vi "UDT_shutdownTest_UserEventsFGV.vi"() -> (3 "Unit Test Framework Results":T1)   [LabVIEW 2017]
doc: "Use this template to create a user-defined test VI. Define your test requirements and wire the results to the <b>Result (Test)</b> control. Do not modify the <b>Unit Test Framework Results</b> indicator."
uses:
  <vilib>/utf/common/utf_test_result_troll.ctl
  <vilib>/utf/common/utf_test_result.ctl
  <vilib>/utf/common/utf_test_result_failure.ctl
  <vilib>/utf/common/utf_test_comparison_operators.ctl
  <vilib>/utf/common/utf_vi_tag.ctl
  RT/UEFGV/Type Def/UEFGV_States.ctl
  <vilib>/Control Software Solutions Ltd/UTF Helper/SubVIs/UTF Boolean Equals.vi
  <vilib>/Control Software Solutions Ltd/UTF Helper/Unit Test Helper.lvlib
  <vilib>/utf/NI_UnitTestFramework.lvlib
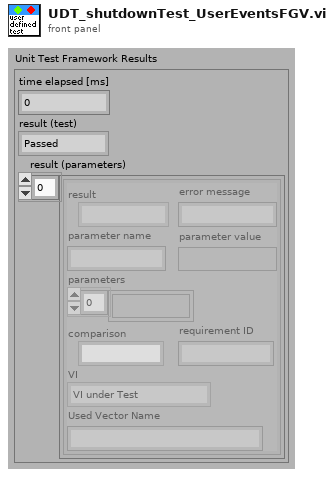
[diagram p1: front panel]
types:
  T1 = typedef "NI_UnitTestFramework.lvlib/utf_test_result_troll.ctl" = cluster{"time elapsed [ms]":u32, "result (test)":T2, "result (parameters)":T3[]}
  T2 = typedef "NI_UnitTestFramework.lvlib/utf_test_result.ctl" = enum16{"Passed", "Failed", "Error", "Skipped", "Not Processed"}
  T3 = typedef "NI_UnitTestFramework.lvlib/utf_test_result_failure.ctl" = cluster{"result":T2, "error message":string, "parameter name":string, "parameter value":variant, "parameters":variant[], "comparison":T4, "requirement ID":string, "VI":T5, "Used Vector Name":string}
  T4 = typedef "NI_UnitTestFramework.lvlib/utf_test_comparison_operators.ctl" = enum16{"=", "!=", ">", ">=", "<", "<=", "range", "symmetric tolerance", "asymmetric tolerance", "string contains", "string not contain", "array size", "string length", "array range", "by element", "array range (limit array)", "user-defined", "array contains", "array not contain", "vector length", "= (elm)", "!= (elm)", "= (case insensitive)", "!= (case insensitive)"}
  T5 = typedef "NI_UnitTestFramework.lvlib/utf_vi_tag.ctl" = enum16{"Setup VI", "VI under Test", "Teardown VI"}
  T6 = typedef "UEFGV_States.ctl" = enum16{"Create", "Get", "Destroy"}
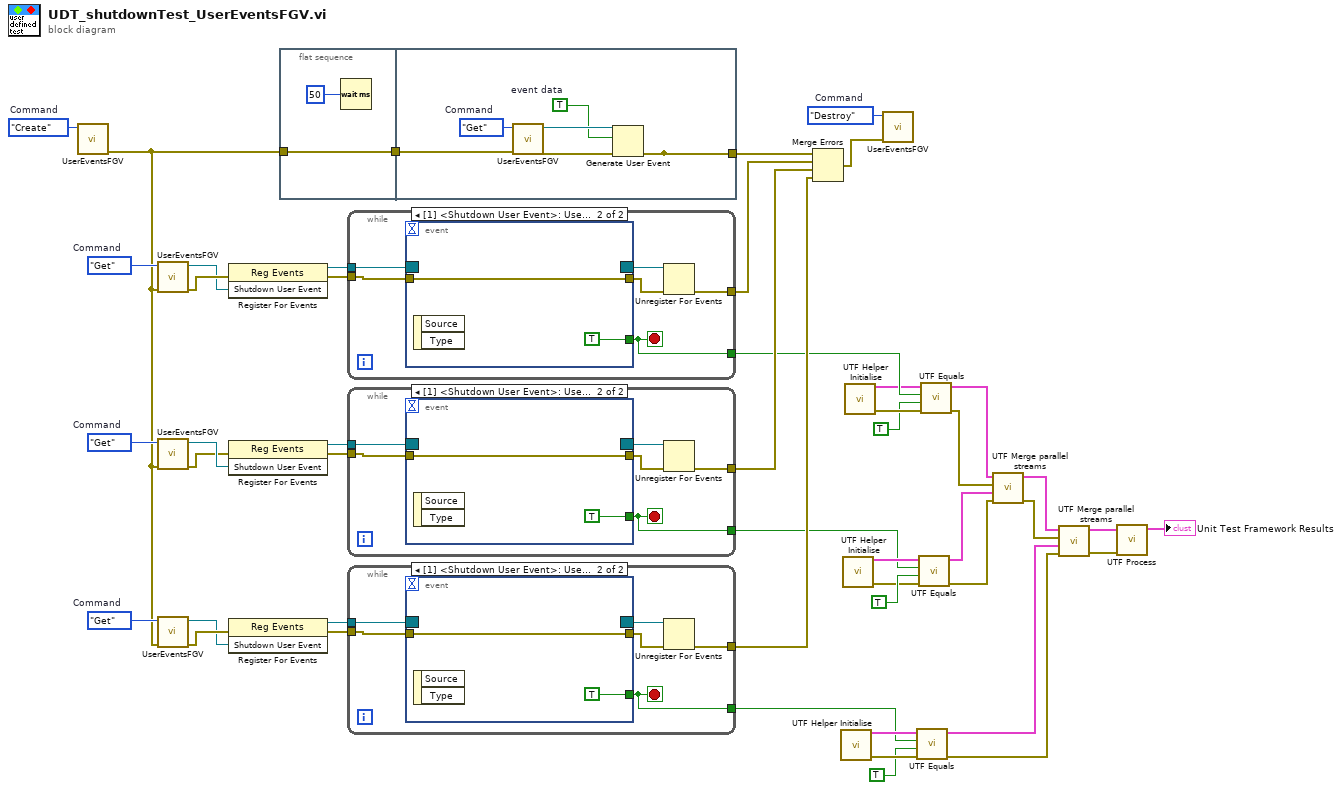
[diagram p0: block diagram]
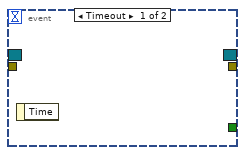
[diagram p2: hidden frame]
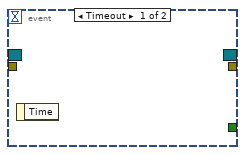
[diagram p3: hidden frame]
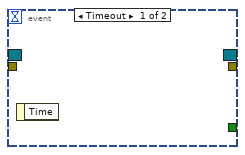
[diagram p4: hidden frame]
diagram:
  w25 = UEFGV_States."Destroy"  # Command
  w35 = UEFGV_States."Get"  # Command
  w36 = UEFGV_States."Get"  # Command
  w45 = UEFGV_States."Get"  # Command
  w47 = UEFGV_States."Create"  # Command
  n1 = call "UserEventsFGV.vi"("Command"=w47) -> ("error out"=w30:errorcluster)  [unwired: 9 in, 1 out]
  n2 = call "UserEventsFGV.vi"("error in (no error)"=w30, "Command"=w45) -> ("error out"=w44:errorcluster, "Shutdown User Event"=w43:refnum<user-event>)  [unwired: 8 in]
  n3 = call "UserEventsFGV.vi"("error in (no error)"=w30, "Command"=w36) -> ("error out"=w37:errorcluster, "Shutdown User Event"=w38:refnum<user-event>)  [unwired: 8 in]
  n4 = call "UserEventsFGV.vi"("error in (no error)"=w30, "Command"=w35) -> ("error out"=w34:errorcluster, "Shutdown User Event"=w33:refnum<user-event>)  [unwired: 8 in]
  n5 = register-events(error in=w44, w43) -> (reference out=w41:refnum<event-registration>, error out=w42:errorcluster)  [unwired: 1 in]
  n6 = register-events(error in=w37, w38) -> (reference out=w40:refnum<event-registration>, error out=w39:errorcluster)  [unwired: 1 in]
  n7 = register-events(error in=w34, w33) -> (reference out=w31:refnum<event-registration>, error out=w32:errorcluster)  [unwired: 1 in]
  n8 = flat-sequence {
    tunnel: [w48] -> w46
    tunnel: w30 -> [w48]
    tunnel: w46 -> [w51]
    tunnel: [w50] -> _
    tunnel: [w50] -> w29
    frame #0 {
      n9 = Wait (ms)(milliseconds to wait=u32 50) -> ()  [unwired: 1 out]
    }
    frame #1 {
      w52 = TRUE  # event data
      w55 = UEFGV_States."Get"  # Command
      n10 = call "UserEventsFGV.vi"("error in (no error)"=w51, "Command"=w55) -> ("error out"=w53:errorcluster, "Shutdown User Event"=w54:refnum<user-event>)  [unwired: 8 in]
      n11 = Generate User Event(user event=w54, event data cluster=w52, error in=w53) -> (error out=w50:errorcluster)  [unwired: 1 in, 1 out]
    }
  }
  n12 = while {
    tunnel: w42 -> [w60]
    tunnel: w41 -> [w61]
    tunnel: [w57] -> w28
    tunnel: [w56] -> w22
    stop <- w56 stop-if-true
    n13 = event shown="[1] <Shutdown User Event>: User Event" {
      selector: w61 -> [_ _]
      dyn-events: [_ _] -> w59
      timeout: _ -> [_ _]
      tunnel: [_ TRUE] -> w56
      tunnel: [_ w62] -> w58
      tunnel: w60 -> [_ w62]
      event Timeout {
        n14 = event-data() -> ()  [unwired: 1 in, 1 out]
      }
      event User Event {
        n15 = event-data() -> ()  [unwired: 1 in, 2 out]
      }
    }
    n16 = Unregister For Events(event registration refnum=w59, error in=w58) -> (error out=w57:errorcluster)
  }
  n17 = while {
    tunnel: w39 -> [w68]
    tunnel: w40 -> [w69]
    tunnel: [w65] -> w26
    tunnel: [w64] -> w15
    stop <- w64 stop-if-true
    n18 = event shown="[1] <Shutdown User Event>: User Event" {
      selector: w69 -> [_ _]
      dyn-events: [_ _] -> w67
      timeout: _ -> [_ _]
      tunnel: [_ TRUE] -> w64
      tunnel: [_ w70] -> w66
      tunnel: w68 -> [_ w70]
      event Timeout {
        n19 = event-data() -> ()  [unwired: 1 in, 1 out]
      }
      event User Event {
        n20 = event-data() -> ()  [unwired: 1 in, 2 out]
      }
    }
    n21 = Unregister For Events(event registration refnum=w67, error in=w66) -> (error out=w65:errorcluster)
  }
  n22 = while {
    tunnel: w32 -> [w76]
    tunnel: w31 -> [w77]
    tunnel: [w73] -> w27
    tunnel: [w72] -> w11
    stop <- w72 stop-if-true
    n23 = event shown="[1] <Shutdown User Event>: User Event" {
      selector: w77 -> [_ _]
      dyn-events: [_ _] -> w75
      timeout: _ -> [_ _]
      tunnel: [_ TRUE] -> w72
      tunnel: [_ w78] -> w74
      tunnel: w76 -> [_ w78]
      event Timeout {
        n24 = event-data() -> ()  [unwired: 1 in, 1 out]
      }
      event User Event {
        n25 = event-data() -> ()  [unwired: 1 in, 2 out]
      }
    }
    n26 = Unregister For Events(event registration refnum=w75, error in=w74) -> (error out=w73:errorcluster)
  }
  n27 = Merge Errors(w29, w28, w26, w27) -> (w24:errorcluster)
  n28 = call <vilib>:"UTF Helper Initialise.vi"() -> ("error out"=w13:errorcluster, "results array"=w14:T3[])  [unwired: 10 in]
  n29 = call <vilib>:"UTF Helper Initialise.vi"() -> ("error out"=w17:errorcluster, "results array"=w16:T3[])  [unwired: 10 in]
  n30 = call <vilib>:"UTF Helper Initialise.vi"() -> ("error out"=w20:errorcluster, "results array"=w21:T3[])  [unwired: 10 in]
  n31 = call "UserEventsFGV.vi"("error in (no error)"=w24, "Command"=w25) -> ()  [unwired: 8 in, 2 out]
  n32 = call-poly <vilib>:"UTF Equals.vi"("error in (no error)"=w13, "Test Value"=TRUE, "Input"=w11, "Input Results"=w14) -> ("error out"=w4:errorcluster, "Output Results"=w3:T3[])  [unwired: 6 in]
  n33 = call-poly <vilib>:"UTF Equals.vi"("error in (no error)"=w17, "Test Value"=TRUE, "Input"=w15, "Input Results"=w16) -> ("error out"=w7:errorcluster, "Output Results"=w8:T3[])  [unwired: 6 in]
  n34 = call-poly <vilib>:"UTF Equals.vi"("error in (no error)"=w20, "Test Value"=TRUE, "Input"=w22, "Input Results"=w21) -> ("error out"=w9:errorcluster, "Output Results"=w10:T3[])  [unwired: 6 in]
  n35 = call <vilib>:"UTF Merge parallel streams.vi"("error in 2"=w7, "Results input 2"=w8, "error in 1"=w9, "Results input 1"=w10) -> ("error out"=w5:errorcluster, "Concatenated Results"=w6:T3[])  [unwired: 6 in]
  n36 = call <vilib>:"UTF Merge parallel streams.vi"("error in 2"=w4, "Results input 2"=w3, "error in 1"=w5, "Results input 1"=w6) -> ("error out"=w1:errorcluster, "Concatenated Results"=w2:T3[])  [unwired: 6 in]
  n37 = call <vilib>:"UTF Process.vi"("error in (no error)"=w1, "results array"=w2) -> ("Unit Test Framework Results"=→"Unit Test Framework Results":T1)  [unwired: 9 in]
